vi "BlackDump.vi"() -> ()   [LabVIEW 2010]
uses:
  <vilib>/Waveform/DWDTOps.llb/DWDT Analog to Digital.vi
panel:
  in  "Tab":enum32{"Timegraph", "Logic Table / Export Data"}(tab) caption="Tab Control"
  out "Dumping":bool
  out "Status":bool
  in  "Start Button":bool
  out "Digital Waveform Graph":digitalwaveform(graph)
  in  "ACQ=1/REF=0":bool=TRUE
  in  "Serial Port COM":refnum<visa-resource-name>
  out "IDN":string
  out "End":bool
  in  "ACQ/Start+ACQ":bool=TRUE
  in  "stop":bool
  out "output waveform 3":digitalwaveform(waveform)={"t0"=timestamp(0 s since 1904-01-01), "dt"=1.0, "Y"={"transitions"=[], "data"=[]}}
  out "output waveform 2":digitalwaveform(waveform)={"t0"=timestamp(0 s since 1904-01-01), "dt"=1.0, "Y"={"transitions"=[], "data"=[]}}
  out "output waveform":digitalwaveform(waveform)={"t0"=timestamp(0 s since 1904-01-01), "dt"=1.0, "Y"={"transitions"=[], "data"=[]}}
  out "Debug Error":errorcluster
  out "Memory Dump (DEC)":u32[](array[numeric])
  # "Memory dump only"
  # "Acquisition Memory"
  # "Francesco Liguoro\nV.0.5 \n28/12/18"
  # "Reference Memory"
  # "Start acquisition and view"
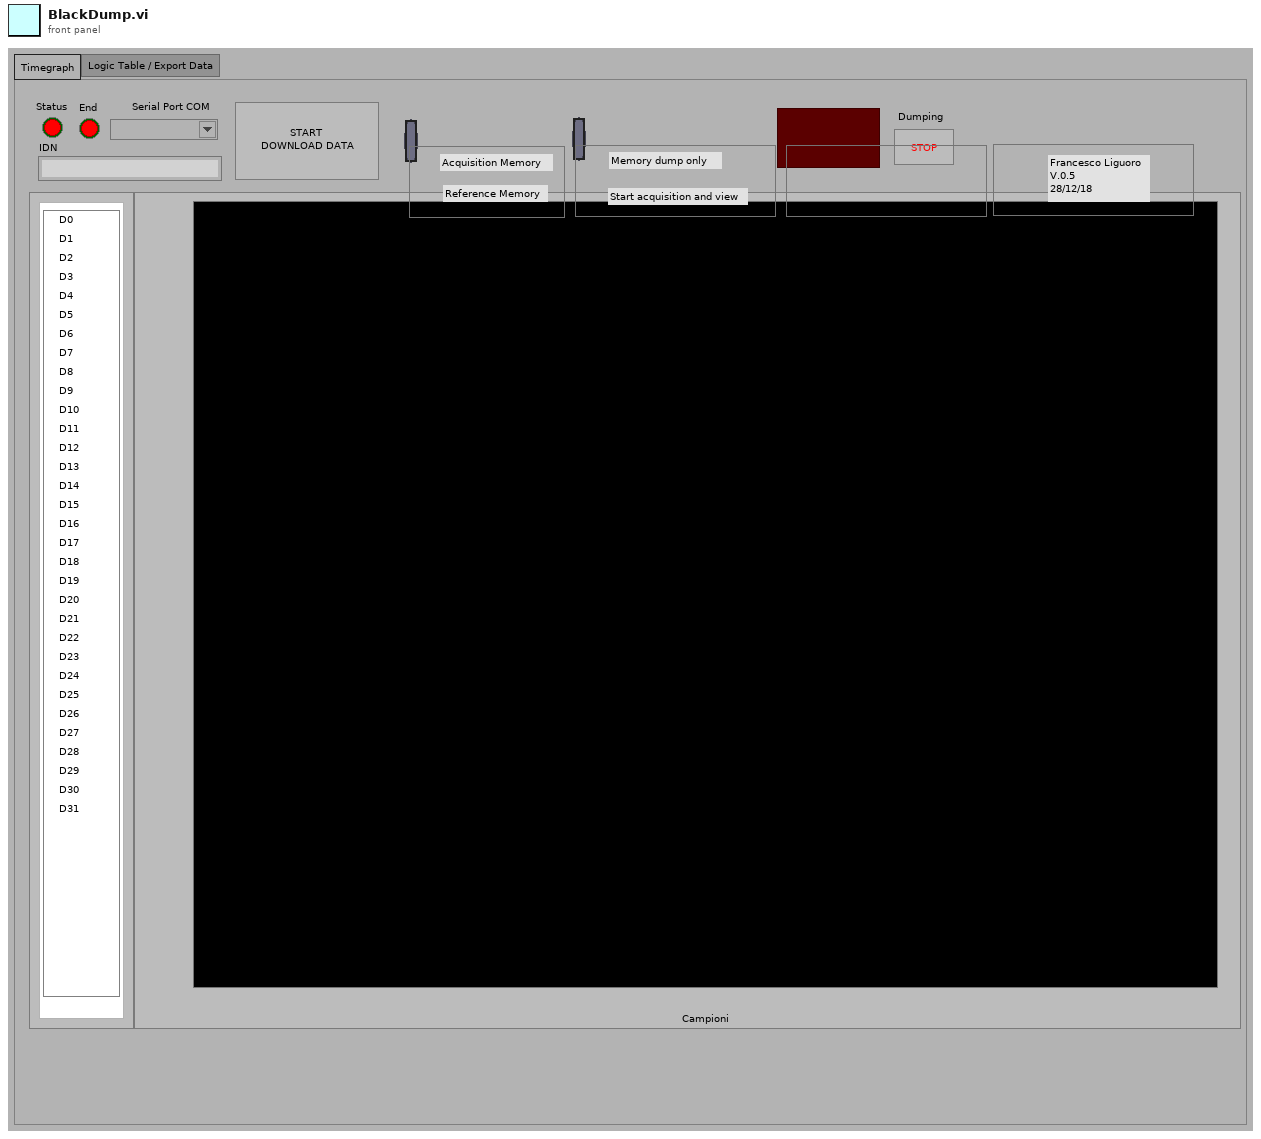
[diagram p1: front panel]
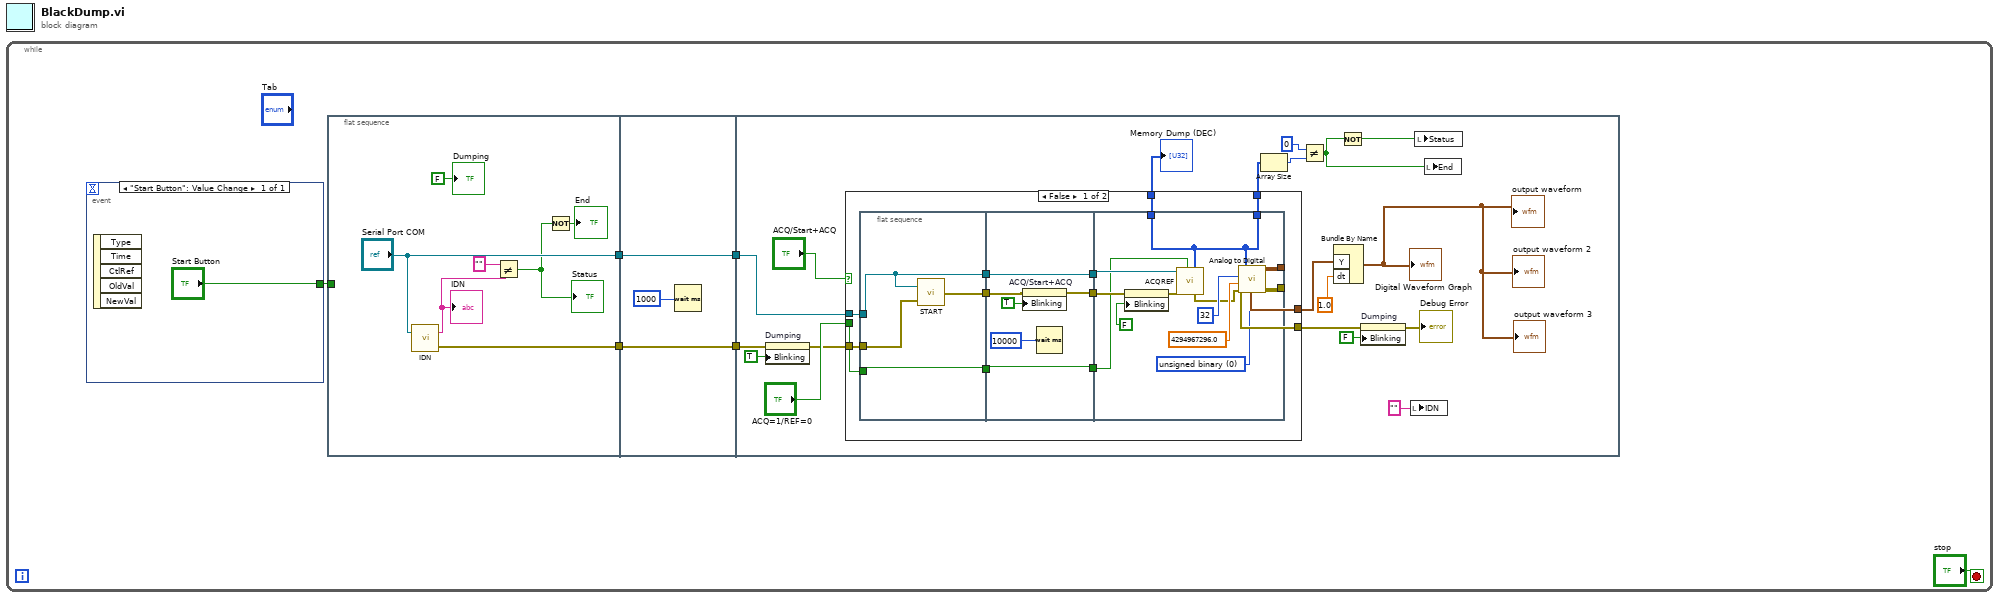
[diagram p0: block diagram]
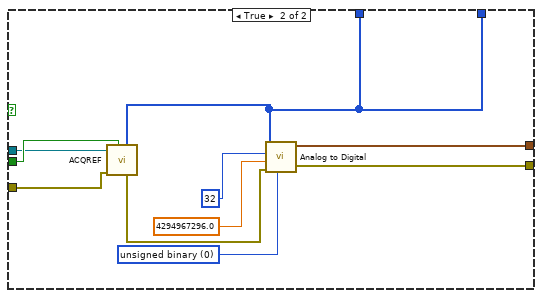
[diagram p2: hidden frame]
diagram:
  n1 = while {
    stop <- "stop" stop-if-true
    n2 = event shown="[0] \"Start Button\": Value Change" {
      selector: _ -> [_]
      dyn-events: _ -> [_]
      timeout: _ -> [_]
      tunnel: ["Start Button"] -> w2
      event "Start Button": Value Change {
        n3 = event-data() -> ()  [unwired: 1 in, 5 out]
      }
    }
    n4 = flat-sequence {
      tunnel: ["Serial Port COM"] -> w6
      tunnel: [w13] -> w5
      tunnel: w2 -> [_]
      tunnel: w6 -> [w17]
      tunnel: [w17] -> w4
      tunnel: [w16] -> w3
      tunnel: w5 -> [w16]
      tunnel: w4 -> [w33]
      tunnel: w3 -> [w22]
      frame #0 {
        n5 = call "IDN.vi"("VISA resource name"="Serial Port COM") -> ("error out"=w13:errorcluster, "IDN"=w12:string)  [unwired: 1 in]
        "IDN" <- w12
        n6 = Not Equal?(x="", y=w12) -> (x != y?=w10:bool)
        "Status" <- w10
        n7 = Not(x=w10) -> (.not. x?=→"End":bool)
        "Dumping" <- FALSE ("Dumping")
      }
      frame #1 {
        n8 = Wait (ms)(milliseconds to wait=u32 1000) -> ()  [unwired: 1 out]
      }
      frame #2 {
        n9 = property on="Dumping" class="Bool (strict)"(error in=w22, "Blinking"=TRUE) -> (error out=w23:errorcluster)  [unwired: 1 in, 1 out]
        n10 = case shown="False" "ACQ/Start+ACQ" {
          tunnel: "ACQ=1/REF=0" -> [w45 w74]
          tunnel: [w48 w81] -> w19
          tunnel: [w49 w79] -> w34
          tunnel: w33 -> [w44 w73]
          tunnel: w23 -> [w41 w76]
          tunnel: [w37 w72] -> w28
          tunnel: [w38 w72] -> w27
          frame False {
            n11 = flat-sequence {
              tunnel: [w53] -> w46
              tunnel: w45 -> [w53]
              tunnel: w44 -> [w52]
              tunnel: [w52] -> w43
              tunnel: w41 -> [w51]
              tunnel: [w50] -> w39
              tunnel: [w59] -> w47
              tunnel: w46 -> [w59]
              tunnel: w43 -> [w58]
              tunnel: [w58] -> w42
              tunnel: [w54] -> w40
              tunnel: w39 -> [w55]
              tunnel: [w68] -> w49
              tunnel: [w67] -> w48
              tunnel: w47 -> [w62]
              tunnel: w42 -> [w63]
              tunnel: w40 -> [w65]
              tunnel: [w61] -> w38
              tunnel: [w61] -> w37
              frame #0 {
                n12 = call "START.vi"("error in (no error)"=w51, "VISA resource name"=w52) -> ("error out"=w50:errorcluster)
              }
              frame #1 {
                n13 = property on="ACQ/Start+ACQ" class="Bool (strict)"(error in=w55, "Blinking"=TRUE) -> (error out=w54:errorcluster)  [unwired: 1 in, 1 out]
                n14 = Wait (ms)(milliseconds to wait=u32 10000) -> ()  [unwired: 1 out]
              }
              frame #2 {
                w69 = u16 0 items=["unsigned binary", "offset binary", "2's complement"] ("data format (offset binary)")
                n15 = property on="ACQ/Start+ACQ" class="Bool (strict)"(error in=w65, "Blinking"=FALSE) -> (error out=w64:errorcluster)  [unwired: 1 in, 1 out]
                n16 = call "ACQREF.vi"("ACQ=1/REF=0"=w62, "error in (no error)"=w64, "VISA resource name"=w63) -> ("error out"=w60:errorcluster, "Number_array"=w61:u32[])  [unwired: 3 in, 4 out]
                n17 = call-poly <vilib>:"Analog to Digital.vi"("data format (offset binary)"=w69, "error in (no error)"=w60, "full-scale range (pk-pk)"=4294967296.0, "resolution (16 bit)"=32, "analog waveform"=w61) -> ("error out"=w67:errorcluster, "digital waveform"=w68:digitalwaveform)  [unwired: 3 in, 2 out]
              }
            }
          }
          frame True {
            w80 = u16 0 items=["unsigned binary", "offset binary", "2's complement"] ("data format (offset binary)")
            n18 = call "ACQREF.vi"("ACQ=1/REF=0"=w74, "error in (no error)"=w76, "VISA resource name"=w73) -> ("error out"=w75:errorcluster, "Number_array"=w72:u32[])  [unwired: 3 in, 4 out]
            n19 = call-poly <vilib>:"Analog to Digital.vi"("data format (offset binary)"=w80, "error in (no error)"=w75, "full-scale range (pk-pk)"=4294967296.0, "resolution (16 bit)"=32, "analog waveform"=w72) -> ("error out"=w81:errorcluster, "digital waveform"=w79:digitalwaveform)  [unwired: 3 in, 2 out]
          }
        }
        "Memory Dump (DEC)" <- w28
        n20 = Array Size(array=w27) -> (size(s)=w32:i32)
        n21 = Not Equal?(x=0, y=w32) -> (x != y?=w30:bool)
        n22 = Bundle By Name("Y"=w34, "dt"=1.0) -> (→"Digital Waveform Graph" →"output waveform" →"output waveform 2" →"output waveform 3":digitalwaveform)  [unwired: 1 in]
        n23 = Not(x=w30) -> (.not. x?=w29:bool)
        n24 = property on="Dumping" class="Bool (strict)"(error in=w19, "Blinking"=FALSE) -> (error out=→"Debug Error":errorcluster)  [unwired: 1 in, 1 out]
        n25 = local write "IDN"("" ("IDN")) -> ()
        n26 = local write "Status"(w29) -> ()
        n27 = local write "End"(w30) -> ()
      }
    }
  }
